vi "车牌号识别.vi"() -> ()   [LabVIEW 2018]
uses:
  <vilib>/userdefined/High Color/IMAQdx.ctl
  <vilib>/vision/NI_Vision_Development_Module.lvlib
  <vilib>/vision/driver/NI_Vision_Acquisition_Software.lvlib
panel:
  in  "停止":bool
  out "Read String":string
  out "Image":T1(plugin-control)
  in  "Rectangle":T2 {"Rotation" min=-90.0 max=90.0 step=1.0 format="%.2f"; "Left" scale=0.0..1024.0; "Right" scale=0.0..1024.0}
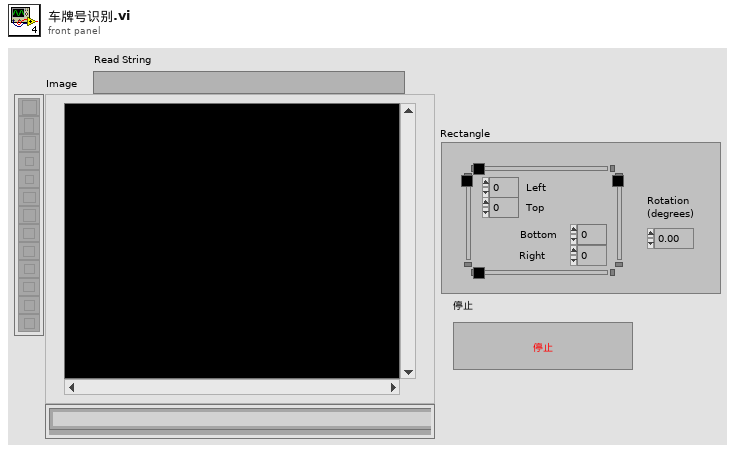
[diagram p1: front panel]
types:
  T1 = typedef "IMAQ Image.ctl" = refnum<image>
  T2 = typedef "IMAQ Rectangle" = cluster{"Left":i32, "Top":i32, "Right":i32, "Bottom":i32, "Rotation":dbl}
  T3 = typedef "IMAQdx.ctl" = refnum<k21>
  T4 = typedef "IMAQ OCR Session.ctl" = refnum<k1>
  T5 = typedef "ROI Descriptor" = cluster{"Global Rectangle":i32[], "Contours":cluster{"ID":enum32{"External", "Internal"}, "Type":u32, "Coordinates":i32[]}[]}
  T6 = cluster{"Global Rectangle":i32[], "Contours":cluster{"ID":enum32{"External", "Internal"}, "Type":u32, "Coordinates":i32[]}[]}
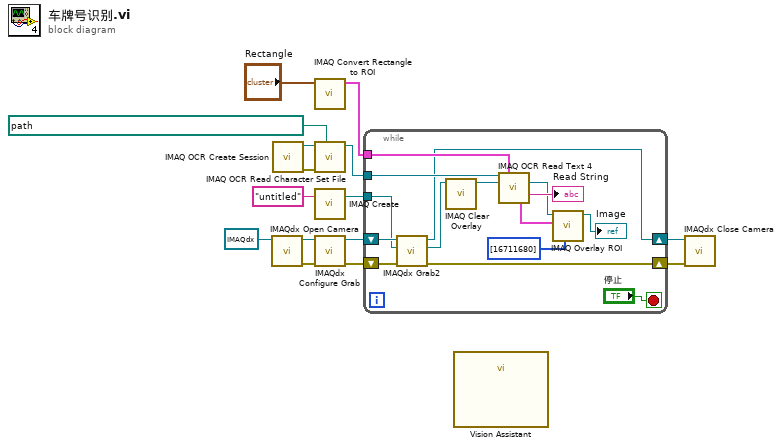
[diagram p0: block diagram]
diagram:
  n1 = call <vilib>:"IMAQdx Open Camera.vi"("Session In"=T3 refnum) -> ("error out"=w6:errorcluster, "Session Out"=w7:T3)  [unwired: 9 in]
  n2 = call "IMAQ OCR Create Session"() -> ("error out"=w13:errorcluster, "IMAQ OCR Session"=w12:T4)  [unwired: 10 in]
  n3 = call "IMAQ Convert Rectangle to ROI"("Rectangle"="Rectangle") -> ("ROI Descriptor"=w9:T5)  [unwired: 8 in, 1 out]
  n4 = call "IMAQ OCR Read Character Set File"("File Path"=path "D:/Labviewprogram/视觉/车牌号识别/车牌号3.abc", "error in (no error)"=w13, "IMAQ OCR Session"=w12) -> ("IMAQ OCR Session (dup)"=w10:T4)  [unwired: 6 in, 2 out]
  n5 = call "IMAQ Create"("Image Name"="untitled") -> ("New Image"=w14:T1)  [unwired: 4 in, 1 out]
  n6 = call <vilib>:"IMAQdx Configure Grab.vi"("error in"=w6, "Session In"=w7) -> ("error out"=w3:errorcluster, "Session Out"=w4:T3)  [unwired: 8 in]
  n7 = while {
    shift-right: [w16] -> w2
    shift-left: w4 -> [w21]
    shift-right: [w18] -> w1
    shift-left: w3 -> [w19]
    tunnel: w14 -> [w20]
    tunnel: w10 -> [w30]
    tunnel: w9 -> [w29]
    stop <- "停止" stop-if-true
    n8 = call <vilib>:"IMAQdx Grab2.vi"("error in"=w19, "Image In"=w20, "Session In"=w21) -> ("error out"=w18:errorcluster, "Image Out"=w17:T1, "Session Out"=w16:T3)  [unwired: 5 in, 1 out]
    n9 = call "IMAQ Clear Overlay"("Image"=w17) -> ("Image Out"=w22:T1)  [unwired: 9 in, 1 out]
    n10 = call "IMAQ OCR Read Text 4"("IMAQ OCR Session"=w30, "ROI Descriptor"=w29, "Image"=w22) -> ("Image (dup)"=w25:T1, "Read String"=→"Read String":string, "ROI Bounding Characters"=w26:T6)  [unwired: 6 in, 4 out]
    n11 = call "IMAQ Overlay ROI"("Colors (Green)"=u32[] [16711680], "ROI Descriptor"=w26, "Image"=w25) -> ("Image Out"=→"Image":T1)  [unwired: 7 in, 1 out]
  }
  n12 = call "Vision Assistant"() -> ()  [unwired: 12 in]
  n13 = call <vilib>:"IMAQdx Close Camera.vi"("error in"=w1, "Session In"=w2) -> ()  [unwired: 9 in, 1 out]
